vi "Set Variables.vi"(8 "error in (no error)":errorcluster, 10 "Variables":variant, 11 "Message Popup in":refnum<class "Statement.lvclass">) -> (0 "error out":errorcluster, 3 "Message Popup out":refnum<class "Statement.lvclass">)   [LabVIEW 2019, in "Statement.lvclass"]
uses:
  Statement.lvclass
  Statement.lvclass/Statement.ctl
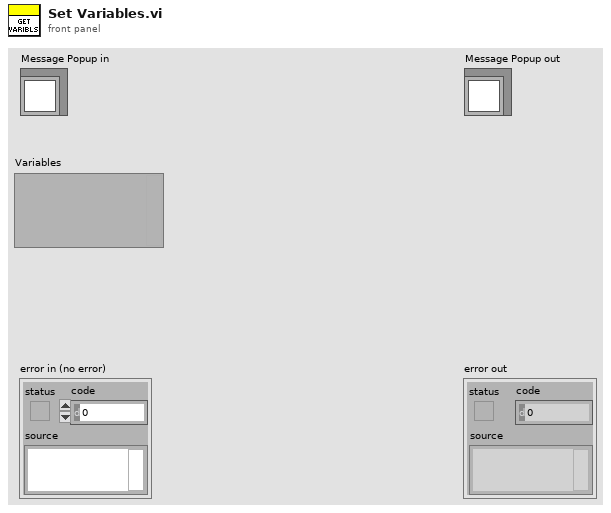
[diagram p1: front panel]
types:
  T1 = typedef "Statement.lvclass/Variables.ctl" = cluster{"leftoperand":string, "rightoperand":variant}
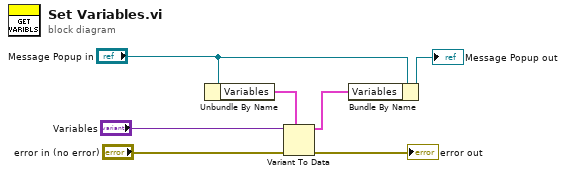
[diagram p0: block diagram]
diagram:
  n1 = Unbundle By Name("Message Popup in") -> ("Variables"=w2:T1)
  n2 = Variant To Data(error in="error in (no error)", type=w2, Variant="Variables") -> (data=w1:T1, error out=→"error out":errorcluster)
  n3 = Bundle By Name(cluster="Message Popup in", "Variables"=w1) -> (→"Message Popup out":refnum<class "Statement.lvclass">)
